vi "Cnvrt Y SI units.vi"(0 "reference in":refnum<class "XYgraph.lvclass">, 2 "Units (micro)":T1="micro", 3 "Offset":dbl, 5 "error in (no error)":errorcluster) -> (14 "reference out":refnum<class "XYgraph.lvclass">, 19 "error out":errorcluster)   [LabVIEW 2019, in "XYgraph.lvclass"]
doc: "Changes the SI units of an X axis"
uses:
  XYgraph.lvclass
  Units --enum.ctl
  <vilib>/Utility/miscctls.llb/LVOffsetAndMultiplierTypeDef.ctl
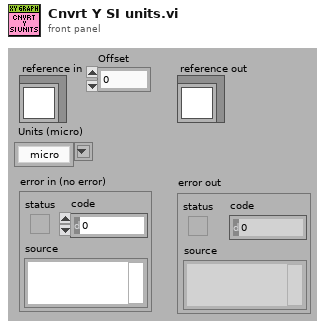
[diagram p1: front panel]
types:
  T1 = typedef "XYgraph.lvclass/Units --enum.ctl" = string
  T2 = typedef "LVOffsetAndMultiplierTypeDef.ctl" = cluster{"Offset":dbl, "Multiplier":dbl}
  T3 = typedef "XYgraph.lvclass/ObjectAttributes.ctl" = cluster{"FPref":T4, "MyAttribute":dbl, "X multiplier":dbl, "Y multiplier":dbl, "X Scale name":string, "Y Scale name":string, "Fcurve metadata":T5, "Fcurve":refnum<class "Fcurve.lvclass">}
  T4 = typedef "XYgraph.lvclass/XY graph ref.ctl" = refnum<vi>
  T5 = typedef "Fcurve.lvclass/Metadata.ctl" = cluster{"dt (us)":dbl, "Dec Factor":dbl, "Z piezo Sensitivity (nm/V)":dbl, "K (N/m)":dbl, "Sp (V)":dbl, "Contact (ms)":dbl, "Zpos contact":dbl, "Vel_app (nm/s)":dbl, "Vel_ret (nm/s)":dbl, "deltaV (nm)":dbl, "Def_V0 (v)":dbl, "Piezo gain":dbl, "invOLS (nm/V)":dbl}
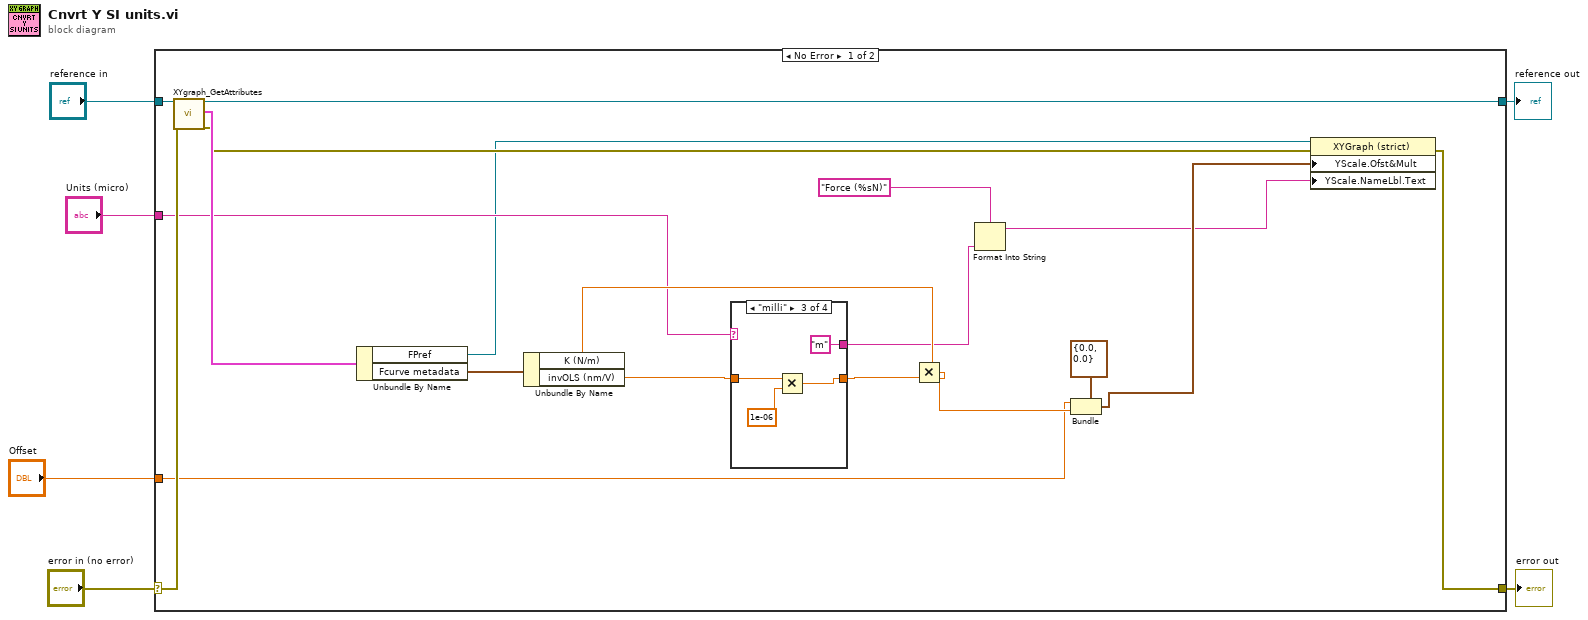
[diagram p0: block diagram]
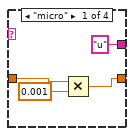
[diagram p2: hidden frame]
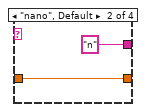
[diagram p3: hidden frame]
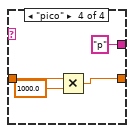
[diagram p4: hidden frame]
diagram:
  n1 = case shown="No Error" "error in (no error)" {
    selector: "error in (no error)" -> [w25 w41]
    tunnel: [w17 w41] -> w5
    tunnel: [w9 w40] -> w3
    tunnel: "reference in" -> [w24 w40]
    tunnel: "Units (micro)" -> [w18 _]
    tunnel: "Offset" -> [w11 _]
    frame No Error {
      n2 = call "XYgraph_GetAttributes.vi"("reference in"=w24, "error in (no error)"=w25) -> ("reference out"=w9:refnum<class "XYgraph.lvclass">, "attributes"=w19:T3, "error out"=w8:errorcluster)  [unwired: 14 in, 1 out]
      n3 = Unbundle By Name(w19) -> ("FPref"=w7:T4, "Fcurve metadata"=w10:T5)
      n4 = Unbundle By Name(w10) -> ("K (N/m)"=w22:dbl, "invOLS (nm/V)"=w15:dbl)
      n5 = case shown="\"milli\"" w18 {
        tunnel: w15 -> [w29 w31 w35 w39]
        tunnel: [w28 w31 w34 w38] -> w14
        tunnel: ["u" ("input 1") "n" ("input 1") "m" ("input 1") "p" ("input 1")] -> w16
        frame "micro" {
          n6 = Multiply(x=w29, y=0.001) -> (x*y=w28:dbl)
        }
        frame "nano", Default {
        }
        frame "milli" {
          n7 = Multiply(x=w35, y=1e-06) -> (x*y=w34:dbl)
        }
        frame "pico" {
          n8 = Multiply(x=w39, y=1000.0) -> (x*y=w38:dbl)
        }
      }
      n9 = Multiply(x=w22, y=w14) -> (x*y=w20:dbl)
      n10 = Format Into String(format string="Force (%sN)" ("Y Scale.Name Label.Text"), w16) -> (resulting string=w12:string)  [unwired: 2 in, 1 out]
      n11 = Bundle(cluster=T2 {"Offset"=0.0, "Multiplier"=0.0} ("Y Scale.Offset and Multiplier"), "Offset"=w11, "Multiplier"=w20) -> (w21:T2)
      n12 = property on="Property Node" class="XYGraph (strict)"(reference=w7, error in=w8, "YScale.Ofst&Mult"=w21, "YScale.NameLbl.Text"=w12) -> (error out=w17:errorcluster)  [unwired: 1 out]
    }
    frame Error {
    }
  }
  "error out" <- w5
  "reference out" <- w3
